vi "G#BaseTemplateG3_SetModifiedClassAttributes.vi"(0 "reference in":refnum<class "G#BaseTemplateG3.lvclass">, 2 "attributes":T1, 3 "Only unlock data? (F)":bool, 4 "Unlock data if error? (T)":bool=TRUE, 5 "error in (no error)":errorcluster, 7 "Update data even if error? (F)":bool) -> (14 "reference out":refnum<class "G#BaseTemplateG3.lvclass">, 19 "error out":errorcluster)   [LabVIEW 2020, in "G#BaseTemplateG3.lvclass"]
doc: "This VI overwrites the attributes associated with the object reference and unlocks it for write access. If error in is set, the object is unlocked but its data will not be modified.\n\nIn order to use this VI, you must first successfully lock the object's data using this class GetAttributesToModify VI."
uses:
  <vilib>/addons/_AddQ/G#Templates/G#BaseTemplateG3/G#BaseTemplateG3.lvclass
  <vilib>/addons/_AddQ/G#Templates/G#BaseTemplateG3/protected/ClassAttributes.ctl
  <vilib>/addons/_AddQ/G#Templates/G#BaseTemplateG3/G#BaseTemplateG3.lvclass/G#BaseTemplateG3.ctl
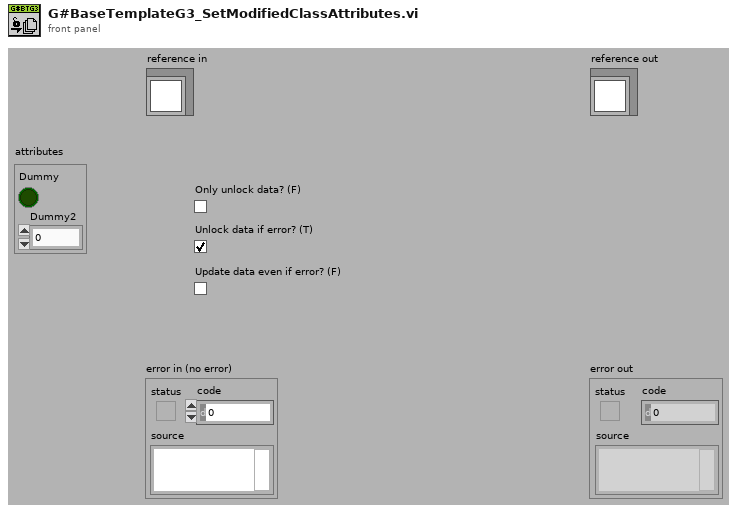
[diagram p1: front panel]
types:
  T1 = typedef "G#BaseTemplateG3.lvclass/ClassAttributes.ctl" = cluster{"Dummy":bool, "Dummy2":dbl}
  T2 = typedef "G#BaseTemplateG3.lvclass/ClassAttributesRef.ctl" = refnum<data-value>
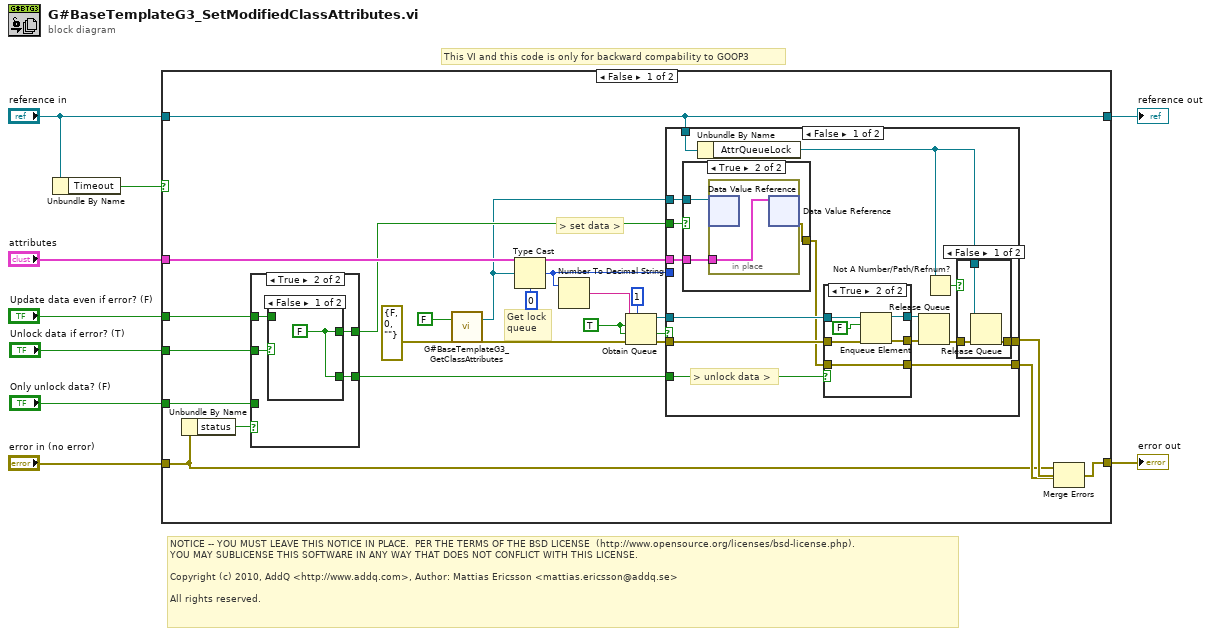
[diagram p0: block diagram]
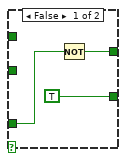
[diagram p2: hidden frame]
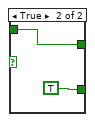
[diagram p3: hidden frame]
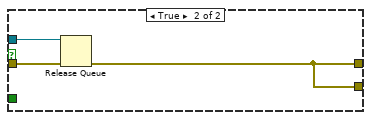
[diagram p7: hidden frame]
diagram:
  # "NOTICE -- YOU MUST LEAVE THIS NOTICE IN PLACE.  PER THE TERMS OF THE BSD LICENSE  (http://www.opensource.org/licenses/bsd-license.php).\nYOU MAY SUBLICENSE THIS SOFTWARE IN ANY WAY THAT DOES NOT CONFLICT WITH THIS LICENSE.\n\nCopyright (c) 2010, AddQ <http://www.addq.com>, Author: Mattias Ericsson <mattias.ericsson@addq.se>\n\nAll rights reserved."
  # "This VI and this code is only for backward compability to GOOP3"
  n1 = Unbundle By Name("reference in") -> ("Timeout"=w1:bool)
  n2 = case shown="False" w1 {
    tunnel: "attributes" -> [w26 _]
    tunnel: [w25 w79] -> w8
    tunnel: "error in (no error)" -> [w12 w79]
    tunnel: "Only unlock data? (F)" -> [w23 _]
    tunnel: "Unlock data if error? (T)" -> [w20 _]
    tunnel: "Update data even if error? (F)" -> [w19 _]
    tunnel: "reference in" -> [w16 w80]
    tunnel: [w16 w80] -> w2
    frame False {
      w32 = TRUE ("create if not found? (T)")
      # "Get lock\nqueue"
      # "> set data >"
      n3 = Unbundle By Name(w12) -> ("status"=w24:bool)
      n4 = case shown="True" w24 {
        tunnel: [w34 w39] -> w22
        tunnel: w23 -> [w36 _]
        tunnel: [TRUE w38] -> w21
        tunnel: w20 -> [_ w40]
        tunnel: w19 -> [_ w37]
        frame False {
          n5 = Not(x=w36) -> (.not. x?=w34:bool)
        }
        frame True {
          n6 = case shown="False" w40 {
            tunnel: [w41 w42] -> w39
            tunnel: [w41 TRUE] -> w38
            tunnel: w37 -> [_ w42]
            frame False {
              w41 = FALSE
            }
            frame True {
            }
          }
        }
      }
      n7 = call <vilib>:"G#BaseTemplateG3_GetClassAttributes.vi"("return data? (T)"=FALSE ("return data"), "error in (no error)"=errorcluster {"status"=FALSE, "code"=0, "source"=""}) -> ("class attributes ref"=w13:T2, "error out"=w10:errorcluster)  [unwired: 13 in, 3 out]
      n8 = Type Cast(type=u32 0, x=w13) -> (*(type *) &x=w17:u32)
      n9 = Number To Decimal String(number=w17) -> (decimal integer string=w33:string)  [unwired: 1 in]
      n10 = Obtain Queue(max queue size (-1, unlimited)=1, name (unnamed)=w33, element data type=w32, create if not found? (T)=w32, error in (no error)=w10) -> (queue out=w28:refnum<queue>, created new?=w29:bool, error out=w30:errorcluster)
      n11 = case shown="False" w29 {
        tunnel: w30 -> [w58 w78]
        tunnel: w28 -> [w57 w76]
        tunnel: [w51 w77] -> w27
        tunnel: w17 -> [_ _]
        tunnel: w22 -> [w54 _]
        tunnel: w26 -> [w53 _]
        tunnel: w21 -> [w52 _]
        tunnel: w16 -> [w49 _]
        tunnel: [w47 w77] -> w15
        tunnel: w13 -> [w46 _]
        frame False {
          # "> unlock data >"
          n12 = case shown="True" w54 {
            tunnel: w53 -> [_ w74]
            tunnel: [_ w73] -> w48
            tunnel: w46 -> [_ w72]
            frame False {
            }
            frame True {
              n13 = in-place {
                in-place-border: w74 -> [w75]
                n14 = in-place-dvr #1(w72) -> ()  [unwired: 2 out]
                n15 = in-place-dvr #1(w75) -> (w73:errorcluster)  [unwired: 1 out]
              }
            }
          }
          n16 = Unbundle By Name(w49) -> ("AttrQueueLock"=w45:refnum<queue>)
          n17 = case shown="True" w52 {
            tunnel: w58 -> [w64 w71]
            tunnel: w57 -> [w65 w70]
            tunnel: [w64 w69] -> w56
            tunnel: [w65 w68] -> w55
            tunnel: w48 -> [w63 w66]
            tunnel: [w63 w66] -> w47
            frame False {
            }
            frame True {
              n18 = Enqueue Element(queue=w70, element=FALSE, error in (no error)=w71) -> (queue out=w68:refnum<queue>, error out=w69:errorcluster)  [unwired: 1 in, 1 out]
            }
          }
          n19 = Release Queue(queue=w55, error in (no error)=w56) -> (error out=w50:errorcluster)  [unwired: 1 in, 2 out]
          n20 = Not A Number/Path/Refnum?(number/path/refnum=w45) -> (NaN/Path/Refnum?=w44:bool)
          n21 = case shown="False" w44 {
            tunnel: [w61 w62] -> w51
            tunnel: w50 -> [w60 w62]
            tunnel: w45 -> [w59 _]
            frame False {
              n22 = Release Queue(queue=w59, error in (no error)=w60) -> (error out=w61:errorcluster)  [unwired: 1 in, 2 out]
            }
            frame True {
            }
          }
        }
        frame True {
          n23 = Release Queue(queue=w76, error in (no error)=w78) -> (error out=w77:errorcluster)  [unwired: 1 in, 2 out]
        }
      }
      n24 = Merge Errors(w12, w27, w15) -> (w25:errorcluster)
    }
    frame True {
      # "Timeout!"
    }
  }
  "error out" <- w8
  "reference out" <- w2
